vi "ble_starts_discovery.vi"(8 "error in (no error)":errorcluster, 10 "GAP Discover Mode (Generic)":T1=1 items=["Discover Limited", "Discover Generic", "Discover Observation"], 11 "COM Bluegiga in":refnum<visa-resource-name>) -> (0 "error out":errorcluster, 1 "payload":u8[](array[numeric]), 2 "success?":bool, 3 "COM Bluegiga out":refnum<visa-resource-name>)   [LabVIEW 2017]
uses:
  type_def/gap_discover_mode.ctl
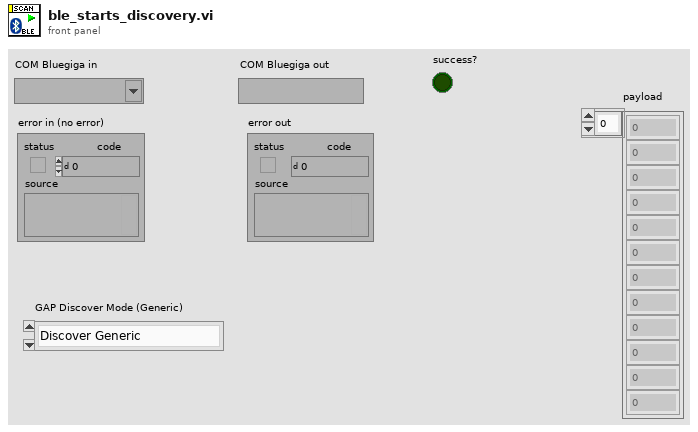
[diagram p1: front panel]
types:
  T1 = typedef "gap_discover_mode.ctl" = u8
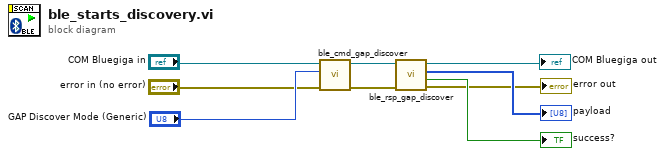
[diagram p0: block diagram]
diagram:
  n1 = call "ble_cmd_gap_discover.vi"("error in (no error)"="error in (no error)", "GAP Discover Mode (Generic)"="GAP Discover Mode (Generic)", "COM Bluegiga in"="COM Bluegiga in") -> ("error out"=w6:errorcluster, "COM Bluegiga out"=w5:refnum<visa-resource-name>)  [unwired: 7 in]
  n2 = call "ble_rsp_gap_discover.vi"("error in (no error)"=w6, "COM Bluegiga in"=w5) -> ("error out"=→"error out":errorcluster, "success?"=→"success?":bool, "full message package"=→"payload":u8[], "COM Bluegiga out"=→"COM Bluegiga out":refnum<visa-resource-name>)  [unwired: 6 in]
